vi "enable_motion.vi"(8 "error in (no error)":errorcluster caption="错误输入（无错误）", 11 "OneMotion 输入":refnum<class "OneMotion.lvclass">) -> (0 "error out":errorcluster caption="错误输出", 3 "OneMotion 输出":refnum<class "OneMotion.lvclass">)   [LabVIEW 2016, in "MotionControl.lvlib" / "OneMotion.lvclass"]
uses:
  <userlib>/MotionControl/OneMotion/OneMotion.lvclass
  <userlib>/MotionControl/OneMotion/OneMotion.lvclass/OneMotion.ctl
  <userlib>/MotionControl/StepMotor/StepMotor.lvclass
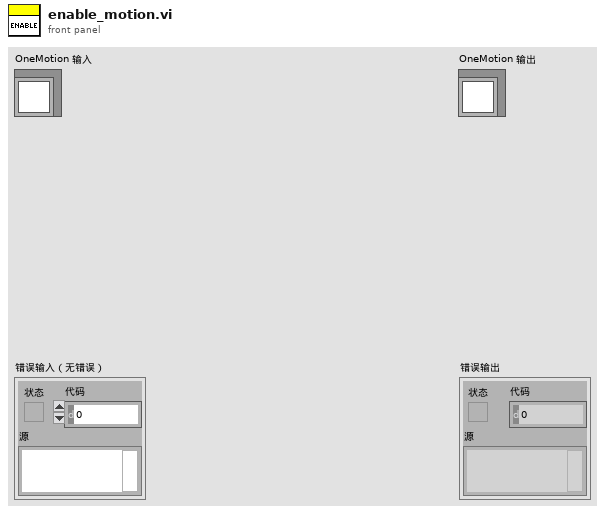
[diagram p1: front panel]
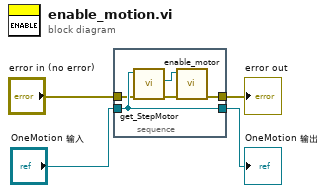
[diagram p0: block diagram]
diagram:
  n1 = stacked-sequence {
    tunnel: [w5] -> w4
    tunnel: [w9] -> w2
    tunnel: "OneMotion 输入" -> [w9]
    tunnel: "error in (no error)" -> [w8]
    frame #0 {
      n2 = call <userlib>:"get_StepMotor.vi"("error in (no error)"=w8, "OneMotion输入"=w9) -> ("error out"=w6:errorcluster, "StepMotor.lvclass"=w7:refnum<class "StepMotor.lvclass">)  [unwired: 7 in, 1 out]
      n3 = call-dynamic "enable_motor.vi"("error in (no error)"=w6, "StepMotor输入"=w7) -> ("error out"=w5:errorcluster)  [unwired: 8 in, 1 out]
    }
  }
  "error out" <- w4
  "OneMotion 输出" <- w2
